vi "Run_Powershell_script.vi"(8 "error in":errorcluster, 11 "Powershell Script":string="$file = \"C:\\Users\\monke\\Desktop\\Work\\VIs to modify\\ONENOTE\\Sandbox\\curl-logo.jpg\"\n\n$read = [convert]::ToBase64String((Get-Content $file -Encoding byte))\n$imageDataURL = [string]::Format(\"data:image/jpeg;base64,{0}\", $read)\n\n$requestBodyPrefix = @\"\n--BlockBoundary\nContent-Disposition:form-data; name=\"Commands\"\nContent-Type:application/json\n\n[{\n\t\"target\": \"body\",\n\t\"action\": \"append\",\n    \"content\": \"<img src=\n\"@\n$requestBodySuffix = @\"\n alt='There is something wrong with the request or the rendering. Please contact Joe'/>\"\n}]\n\n\n--BlockBoundary--\n\"@\n$request1 = $requestBodyPrefix + $imageDataUrl\n$request1 = $request1 + $requestBodySuffix\n$url = 'https://www.onenote.com/api/v1.0/me/notes/pages/0-c8e01dcaf69a4df09e4cc94142adbb9e!47-962DFAE583894FEA!201/content'\n$AccessToken = \"EwAQA61DBAAUcSSzoTJJsy+XrnQXgAKO5cj4yc8AAS6fPc6NVokthrh8Aw3FulD0hYgp7aZyj/mtVLeNARi4RLEL0/Wbr+rQ+0AvAsSRTkAWVMDQenSKh3916rQ85Gi3BaxeKzlXgS3hIOzsyXteoja2swX0Yy/1ucSuS3PDQsNsc6D+dlzpkERiGEPaEM4C//uC08x5ROEVfkqO5qsj9vHtLbpX0ZCKsVCARpgHh/v8EAZ75OQw0wYmVfsnL9pZBkDMYtv+GoWXPRQmR+2Sd7ty0WQ7JFfFKhLPOdTk5IUBzl1KymiBFBgS9/xeWrV0a0XDjUhSpU4molMTKc/7WwM//43cHjzl8+78h4u54CKg21krOqq9f+r7Wj7+KCEDZgAACBFzrI8vXCWb4AGpj4eW2Lohr6Sce8fSAOXqdJUoNi3c03rx/WjvC8HM0K6iV2pp6ODZw2KkXuwMYr1knYE0MKapS2g5jz9CrfvzlP2IFeJrBZMUFsOZMxDYAGs4VPi+ipBSFiX69l16fsZ7e12QBUwcLFCUGZ8x2B/Lvcn8lxNKLhEiPQZyEPufenBbV1NrXOV3uGrJLnypB/BtSZMXIrzFw1zf3mhjKVlKE60mqBBx2ackS+a1LElmOASeBc5IsWqshnYxDx6Hslk910n9RbW0iJZXq5acSUqrxrFIkL1nQlqaeVLaAOUYZBhWDMf7Yzw0/xmUVWAyNHpbud+ZUnDnqpf50evEFonPML6fdW0j+1tVMlltMBvVGTZhy7S3UYrWEmmFAi8ET9mm7AtAc1M9rkCdg6uWeDUeb3ydVOJuExCN5rarazj6+Akimov2ol+wPBWL8NLKzHNpS0c9FTQxypnvwGHenvEnOM78Zl4/IgorEos1yHjfGAkSXp2d7QsT9xf+Xba6PbWCfdRvPekCM+6niRDMjU4Eh9kwLdFxilBQRoxF1lEmcg7EAEOMG71Shz/N/SbI+ti0UdK83MN1keRzMkK5hEiNfSd6YfPLQv39MOg60CcCkbLD779TWLQd8k0otHQ5YnMWAg==\"\n$headers = @{\"Authorization\" = \"Bearer \" + $AccessToken}\n\nInvoke-RestMethod -method 'PATCH' -uri $url -Body $request1 -Headers $headers -ContentType 'multipart/form-data; boundary=BlockBoundary'") -> (0 "error out":errorcluster, 2 "standard error":string, 3 "standard output":string)   [LabVIEW 2020, in "Request.lvclass"]
uses:
  Request.lvclass
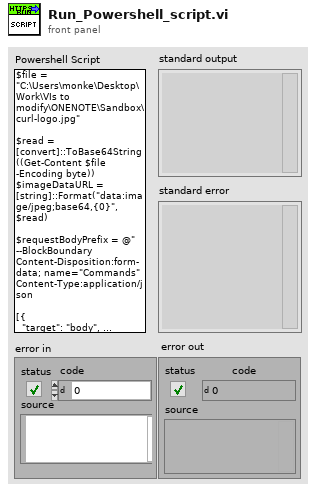
[diagram p1: front panel]
types:
  T1 = enum16{"open", "replace", "create", "open or create", "replace or create", "replace or create with confirmation"}
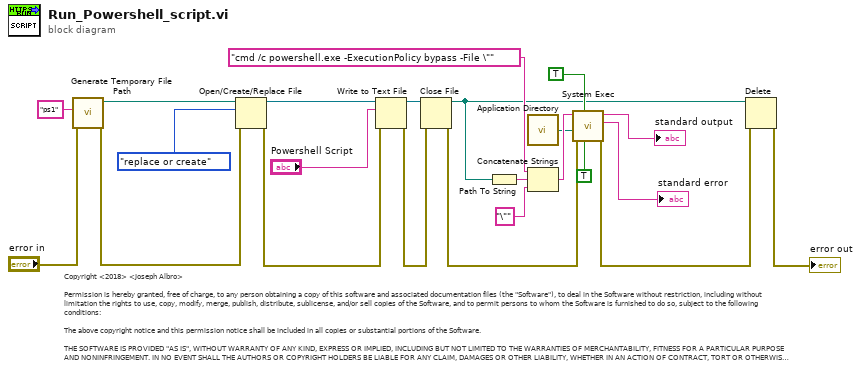
[diagram p0: block diagram]
diagram:
  # "Copyright <2018> <Joseph Albro>\n\nPermission is hereby granted, free of charge, to any person obtaining a copy of this software and associated documentation files (the \"Software\"), to deal in the Software without restriction, including without limitation the rights to use, copy, modify, merge, publish, distribute, sublicense, and/or sell copies of the Software, and to permit persons to whom the Software is furnished to do so, subject to the following conditions:\n\nThe above copyright notice and this permission notice shall be included in all copies or substantial portions of the Software.\n\nTHE SOFTWARE IS PROVIDED \"AS IS\", WITHOUT WARRANTY OF ANY KIND, EXPRESS OR IMPLIED, INCLUDING BUT NOT LIMITED TO THE WARRANTIES OF MERCHANTABILITY, FITNESS FOR A PARTICULAR PURPOSE AND NONINFRINGEMENT. IN NO EVENT SHALL THE AUTHORS OR COPYRIGHT HOLDERS BE LIABLE FOR ANY CLAIM, DAMAGES OR OTHER LIABILITY, WHETHER IN AN ACTION OF CONTRACT, TORT OR OTHERWISE, ARISING FROM, OUT OF OR IN CONNECTION WITH THE SOFTWARE OR THE USE OR OTHER DEALINGS IN THE SOFTWARE."
  n1 = call <vilib>:"Generate Temporary File Path.vi"("error in (no error)"="error in", "Temporary File Extension (tmp)"="ps1") -> ("error out"=w6:errorcluster, "Unique Temporary File Path"=w8:path)  [unwired: 8 in]
  n2 = Open/Create/Replace File(file path (use dialog)=w8, error in=w6, operation (0:open)=T1."replace or create") -> (refnum out=w15:refnum<file>, error out=w13:errorcluster)  [unwired: 3 in, 1 out]
  n3 = Write to Text File(file (use dialog)=w15, text="Powershell Script", error in=w13) -> (refnum out=w14:refnum<file>, error out=w12:errorcluster)  [unwired: 1 in, 1 out]
  n4 = Close File(refnum=w14, error in=w12) -> (path=w1:path, error out=w4:errorcluster)
  n5 = Path To String(path=w1) -> (string=w18:string)
  n6 = call <vilib>:"Application Directory.vi"() -> ("Application Directory"=w2:path)
  n7 = Concatenate Strings("cmd /c powershell.exe -ExecutionPolicy bypass -File \"" ("command line"), w18, "\"" ("string")) -> (w17:string)
  n8 = call <vilib>:"System Exec.vi"("run minimized? (F)"=TRUE, "wait until completion? (T)"=TRUE, "error in (no error)"=w4, "working directory"=w2, "command line"=w17) -> ("error out"=w11:errorcluster, "standard error"=→"standard error":string, "standard output"=→"standard output":string)  [unwired: 3 in, 1 out]
  n9 = Delete(path (use dialog)=w1, error in=w11) -> (error out=→"error out":errorcluster)  [unwired: 3 in, 2 out]
